vi "Get Dependency Nodes.vi"(8 "error in (no error)":errorcluster, 11 "Project XML Editor in":refnum<class "Project XML Editor.lvclass">) -> (0 "error out":errorcluster, 1 "Exist ?":bool, 2 "Dependency Nodes":refnum<k20>[](array[refnum]), 3 "Project XML Editor out":refnum<class "Project XML Editor.lvclass">)   [LabVIEW 2019, in "Project XML Editor.lvclass"]
uses:
  Project XML Editor.lvclass
  <vilib>/xml/Close Reference(Node).vi
  <resource>/objmgr/DOMUserDefRef.rc
  <vilib>/xml/NI_XML.lvlib
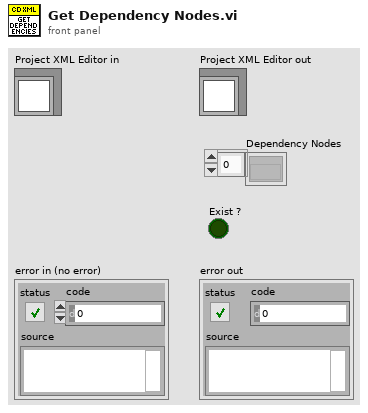
[diagram p1: front panel]
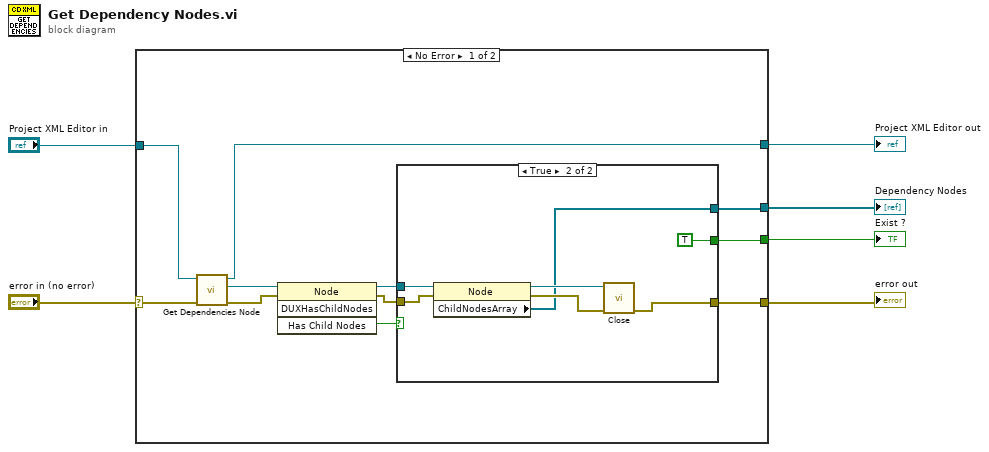
[diagram p0: block diagram]
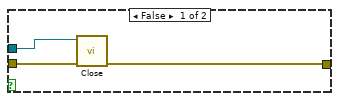
[diagram p2: hidden frame]
diagram:
  n1 = case shown="No Error" "error in (no error)" {
    selector: "error in (no error)" -> [w10 w28]
    tunnel: [w17 w28] -> w6
    tunnel: [w16 w29] -> w5
    tunnel: "Project XML Editor in" -> [w11 w29]
    tunnel: [w8 _] -> w2
    tunnel: [w7 _] -> w1
    frame No Error {
      n2 = call "Get Dependencies Node.vi"("error in (no error)"=w10, "Project XML Editor in"=w11) -> ("error out"=w12:errorcluster, "Dependencies out"=w9:refnum<k20>, "Project XML Editor out"=w16:refnum<class "Project XML Editor.lvclass">)  [unwired: 7 in]
      n3 = invoke class="Node" method="DUXHasChildNodes"(reference=w9, error in=w12) -> (reference out=w15:refnum<k20>, error out=w14:errorcluster, "Has Child Nodes"=w13:bool)  [unwired: 2 in, 1 out]
      n4 = case shown="True" w13 {
        tunnel: w14 -> [w20 w27]
        tunnel: w15 -> [w19 w26]
        tunnel: [w18 w22] -> w17
        tunnel: [_ w23] -> w8
        tunnel: [_ TRUE] -> w7
        frame False {
          n5 = call-poly <vilib>:"Close.vi"("error in (no error)"=w20, "node"=w19) -> ("error out"=w18:errorcluster)  [unwired: 7 in]
        }
        frame True {
          n6 = property class="Node"(reference=w26, error in=w27) -> (reference out=w24:refnum<k20>, error out=w25:errorcluster, "ChildNodesArray"=w23:refnum<k20>[])
          n7 = call-poly <vilib>:"Close.vi"("error in (no error)"=w25, "node"=w24) -> ("error out"=w22:errorcluster)  [unwired: 7 in]
        }
      }
    }
    frame Error {
    }
  }
  "error out" <- w6
  "Project XML Editor out" <- w5
  "Dependency Nodes" <- w2
  "Exist ?" <- w1
